vi "Get Server gRPC UEs.vi"(11 "OOP Server in":refnum<class "HVC3.lvclass">) -> (2 "Server gRPC UEs":T1, 3 "OOP Server out":refnum<class "HVC3.lvclass">)   [LabVIEW 2019, in "HVC3.lvlib" / "HVC3.lvclass"]
uses:
  HVC3.lvclass
  typeDefs/Server gRPC UEs.ctl
  gRPC lvSupport/Server API/typeDefs/gRPCId Cluster.ctl
  gRPC lvSupport/Server API/typeDefs/grpcId.ctl
  HVC3.lvclass/HVC3.ctl
  gRPC lvSupport/gprc-lvsupport.lvlib
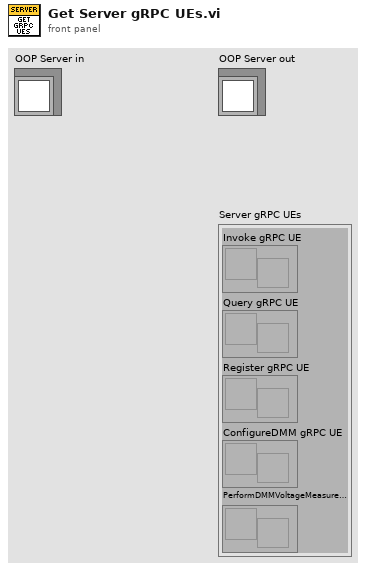
[diagram p1: front panel]
types:
  T1 = typedef "HVC3.lvlib/HVC3.lvclass/Server gRPC UEs.ctl" = cluster{"Invoke gRPC UE":refnum<user-event>, "Query gRPC UE":refnum<user-event>, "Register gRPC UE":refnum<user-event>, "ConfigureDMM gRPC UE":refnum<user-event>, "PerformDMMVoltageMeasurement gRPC UE":refnum<user-event>}
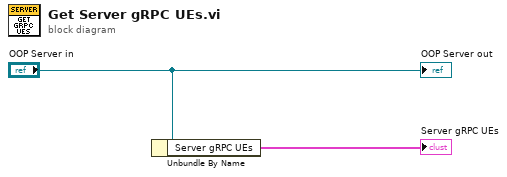
[diagram p0: block diagram]
diagram:
  n1 = Unbundle By Name("OOP Server in") -> ("Server gRPC UEs"=→"Server gRPC UEs":T1)
  "OOP Server out" <- "OOP Server in"
